vi "Init.vi"(8 "error in (no error)":errorcluster, 10 "Size":cluster{"Width":u16, "Height":u16}, 11 "Drawer .Net in":refnum<class "Drawer .Net.lvclass">) -> (0 "error out":errorcluster, 3 "Drawer .Net out":refnum<class "Drawer .Net.lvclass">)   [LabVIEW 2023, in "Glyph .NET Drawer.lvlib" / "Drawer .Net.lvclass"]
uses:
  Drawer .Net.lvclass
  Drawer .Net.lvclass/Drawer .Net.ctl
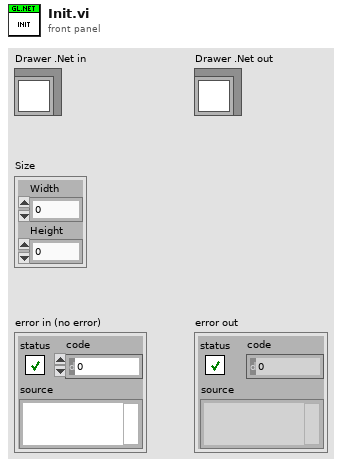
[diagram p1: front panel]
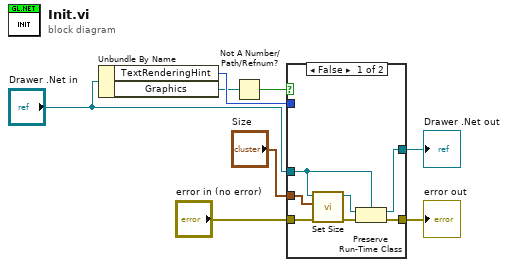
[diagram p0: block diagram]
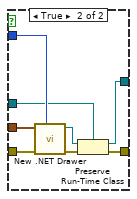
[diagram p2: hidden frame]
diagram:
  n1 = Unbundle By Name("Drawer .Net in") -> ("TextRenderingHint"=w5:i32, "Graphics"=w2:refnum<k24>)
  n2 = Not A Number/Path/Refnum?(number/path/refnum=w2) -> (NaN/Path/Refnum?=w1:bool)
  n3 = case shown="False" w1 {
    tunnel: "Size" -> [w13 w20]
    tunnel: "Drawer .Net in" -> [w9 w16]
    tunnel: [w10 w17] -> w6
    tunnel: w5 -> [_ w23]
    tunnel: "error in (no error)" -> [w15 w22]
    tunnel: [w12 w19] -> w3
    frame False {
      n4 = call "Set Size.vi"("error in (no error)"=w15, "Size"=w13, "Drawer .Net in"=w9) -> ("error out"=w14:errorcluster, "Drawer .Net out"=w11:refnum<class "Drawer .Net.lvclass">)  [unwired: 7 in]
      n5 = Preserve Run-Time Class(object in=w11, error in=w14, 2:w9) -> (object out=w10:refnum<class "Drawer .Net.lvclass">, error out=w12:errorcluster)
    }
    frame True {
      n6 = call "New .NET Drawer.vi"("TextRenderingHint"=w23, "error in (no error)"=w22, "Size"=w20) -> ("error out"=w21:errorcluster, "Canvas out"=w18:refnum<class "Drawer .Net.lvclass">)  [unwired: 7 in]
      n7 = Preserve Run-Time Class(object in=w18, error in=w21, 2:w16) -> (object out=w17:refnum<class "Drawer .Net.lvclass">, error out=w19:errorcluster)
    }
  }
  "error out" <- w3
  "Drawer .Net out" <- w6
